vi "Load Plugin.vi"(6 "timeout (ms)":i32=5000, 8 "error in":errorcluster, 10 "New Plugin":T1, 11 "gRPC ID in":T2) -> (0 "error out":errorcluster, 3 "gRPC ID out":T2)   [LabVIEW 2021, in "CIFManagerClientWrapper.lvlib"]
uses:
  CIFManagerClientWrapper.lvlib
  <vilib>/gRPC/LabVIEW gRPC Library/Shared/grpcId.ctl
  CIFUI/Typedef/New Plugin.ctl
  CIF_Manager_client/RPC Messages/cif_manager_PluginConfig.ctl
  CIF_Manager_client/CIF_Manager_client.lvlib
  <vilib>/gRPC/LabVIEW gRPC Library/grpc-lvsupport-release.lvlib
  CIFUI/CIF_UI.lvclass
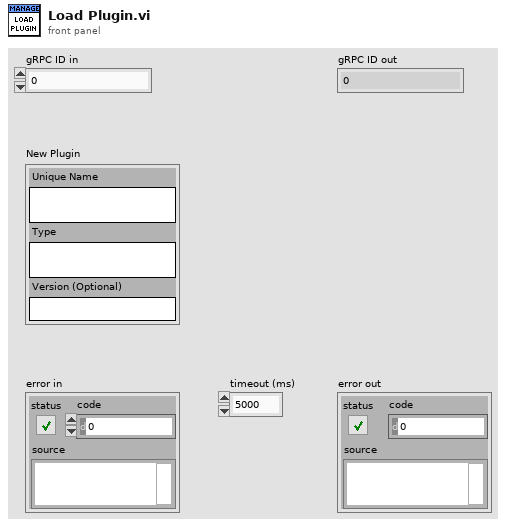
[diagram p1: front panel]
types:
  T1 = typedef "CIF_UI.lvclass/New Plugin.ctl" = cluster{"Unique Name":string, "Type":string, "Version (Optional)":string}
  T2 = typedef "grpc-lvsupport-release.lvlib/grpcId.ctl" = u64
  T3 = typedef "CIF_Manager_client.lvlib/cif_manager_PluginConfig.ctl" = cluster{"plugin_type":string, "plugin_name":string, "version":string}
  T4 = typedef "CIF_Manager_client.lvlib/cif_common_Status.ctl" = cluster{"code":i32, "message":string}
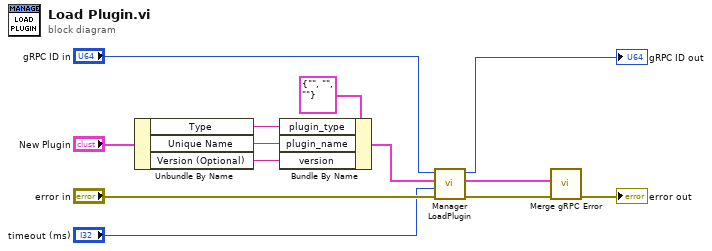
[diagram p0: block diagram]
diagram:
  n1 = Unbundle By Name("New Plugin") -> ("Type"=w3:string, "Unique Name"=w2:string, "Version (Optional)"=w1:string)
  n2 = Bundle By Name(cluster=T3 {"plugin_type"="", "plugin_name"="", "version"=""} ("Plugin"), "plugin_type"=w3, "plugin_name"=w2, "version"=w1) -> (w6:T3)
  n3 = call "Manager LoadPlugin.vi"("error in"="error in", "timeout (ms)"="timeout (ms)", "Request Data"=w6, "gRPC ID"="gRPC ID in") -> ("error out"=w9:errorcluster, "Response Data"=w7:T4, "gRPC ID out"=→"gRPC ID out":T2)  [unwired: 5 in]
  n4 = call "Merge gRPC Error.vi"("error in (no error)"=w9, "gRPC Error"=w7) -> ("error out"=→"error out":errorcluster)  [unwired: 9 in]
